vi "LCP Set Syringe Param.vi"(8 "error in (no error)":errorcluster caption="Fehler (Eingang, kein Fehler)", 9 "Maximum Piston Stroke (mm)":dbl, 10 "Inner Diameter (mm)":dbl, 11 "Pump Handle":i64) -> (0 "error out":errorcluster caption="Fehler (Ausgang)")   [LabVIEW 2023, in "labbCAN_Pump_API.lvlib"]
doc: "LCP_Func long LCP_CALL LCP_SetSyringeParam(dev_hdl hPump,\n double InnerDiameter_mm,\n double MaxPistonStroke_mm);"
uses:
  labbCAN_Pump_API.lvlib
  labbCAN_Pump_API.dll
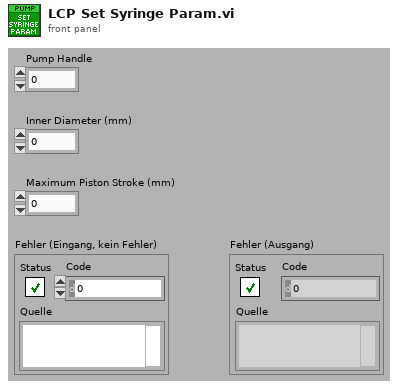
[diagram p1: front panel]
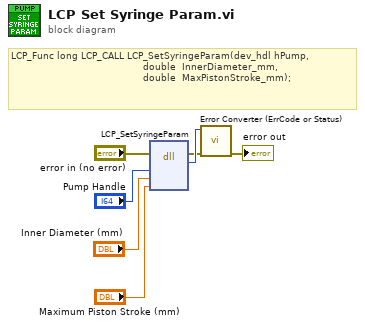
[diagram p0: block diagram]
diagram:
  # "LCP_Func long LCP_CALL LCP_SetSyringeParam(dev_hdl hPump,\n                                            double  InnerDiameter_mm,\n                                            double  MaxPistonStroke_mm);"
  n1 = dll-call lib="C:/GIT/AutomatedSetupAcousticEnergyDensity/CETONI_SDK/labbCAN_Pump_API.*" fn="LCP_SetSyringeParam"(error in="error in (no error)", "hPump"="Pump Handle", "InnerDiameter_mm"="Inner Diameter (mm)", "MaxPistonStroke_mm"="Maximum Piston Stroke (mm)") -> (error out=w2:errorcluster, "Rückgabetyp"=w3:i32)  [unwired: 5 in, 1 out]
  n2 = call "Error Converter (ErrCode or Status).vi"("error in (no error)"=w2, "error code"=w3) -> ("error out"=→"error out":errorcluster)  [unwired: 9 in]
